vi "ExpandTreeAndLinkNodes.vi"(8 "error in (no error)":errorcluster, 10 "ToExpand in":refnum<data-value>, 11 "Tree in":refnum<class "Tree.lvclass">) -> (0 "error out":errorcluster, 1 "ExpandedSearchNodes":refnum<data-value>[](array[refnum]), 2 "ToExpand out":refnum<data-value>, 3 "Tree out":refnum<class "Tree.lvclass">)   [LabVIEW 2010, in "Tree.lvclass"]
doc: "Calls the expand method, and then links the newly expanded nodes. Currently it always links."
uses:
  Tree.lvclass
  TreeNode/TreeNode.lvclass
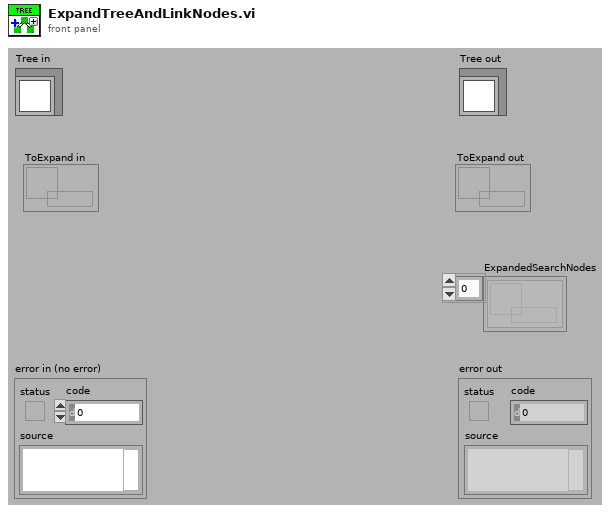
[diagram p1: front panel]
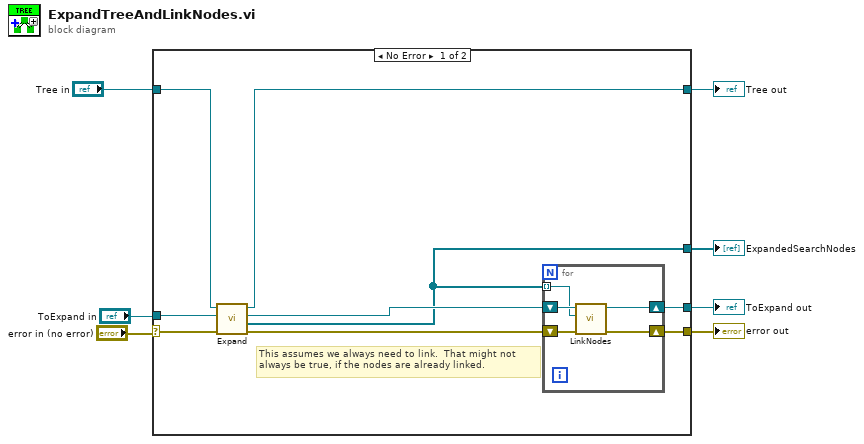
[diagram p0: block diagram]
diagram:
  n1 = case shown="No Error" "error in (no error)" {
    selector: "error in (no error)" -> [w14 w24]
    tunnel: [w16 w24] -> w2
    tunnel: [w15 w23] -> w3
    tunnel: "ToExpand in" -> [w11 w23]
    tunnel: "Tree in" -> [w13 w22]
    tunnel: [w12 w22] -> w6
    tunnel: [w9 _] -> w1
    frame No Error {
      # "This assumes we always need to link.  That might not\nalways be true, if the nodes are already linked."
      n2 = call-dynamic "Expand.vi"("error in (no error)"=w14, "ToExpand in"=w11, "Tree in"=w13) -> ("error out"=w8:errorcluster, "ExpandedSearchNodes"=w9:refnum<data-value>[], "ToExpand out"=w10:refnum<data-value>, "Tree out"=w12:refnum<class "Tree.lvclass">)  [unwired: 5 in]
      n3 = for {
        shift-right: [w19] -> w16
        shift-left: w8 -> [w20]
        tunnel: w9 -> [w18] mode=indexing
        shift-right: [w17] -> w15
        shift-left: w10 -> [w21]
        n4 = call "LinkNodes.vi"("error in (no error)"=w20, "Child in"=w18, "Parent in"=w21) -> ("error out"=w19:errorcluster, "Parent out"=w17:refnum<data-value>)  [unwired: 5 in, 2 out]
      }
    }
    frame Error {
    }
  }
  "error out" <- w2
  "Tree out" <- w6
  "ToExpand out" <- w3
  "ExpandedSearchNodes" <- w1
